vi "ASK.vi"() -> ()   [LabVIEW 2015]
panel:
  out "modulated":dbl[](graph)
  out "carrier":dbl[](graph)
  out "data":i16[](graph)
  in  "Carrier Frequency":dbl
  in  "Numeric":i32
  in  "Sampling Frequency":i32
  in  "data Frequency":dbl
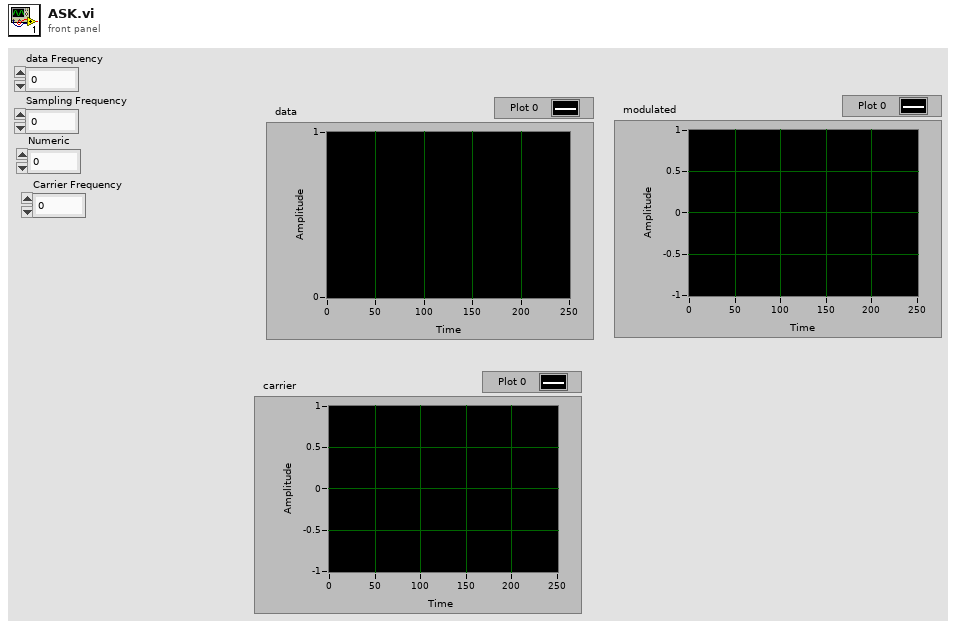
[diagram p1: front panel]
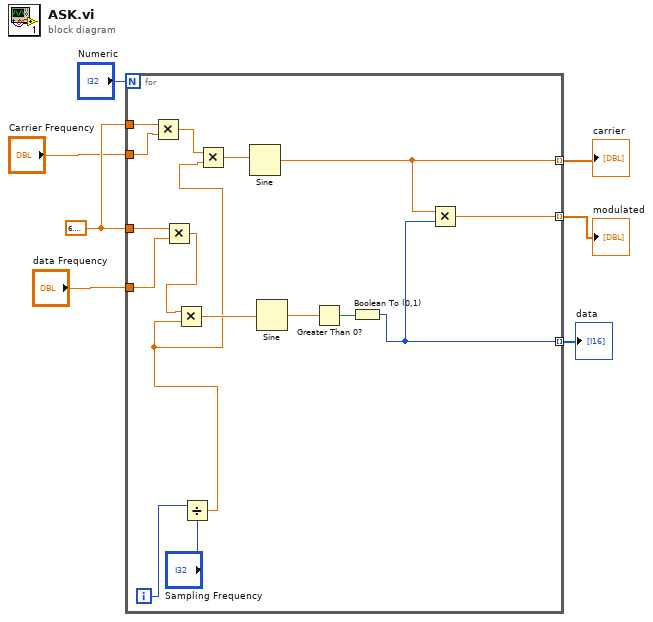
[diagram p0: block diagram]
diagram:
  w5 = 6.283185307179586
  n1 = for {
    N: "Numeric" -> [_]
    tunnel: w5 -> [w23]
    tunnel: "data Frequency" -> [w22]
    tunnel: w5 -> [w17]
    tunnel: "Carrier Frequency" -> [w16]
    tunnel: [w9] -> w3 mode=indexing
    tunnel: [w10] -> w2 mode=indexing
    tunnel: [w8] -> w1 mode=indexing
    i -> [w21]
    n2 = Multiply(x=w17, y=w16) -> (x*y=w15:dbl)
    n3 = Multiply(x=w23, y=w22) -> (x*y=w19:dbl)
    n4 = Divide(x=w21, y="Sampling Frequency") -> (x/y=w14:dbl)
    n5 = Multiply(x=w19, y=w14) -> (x*y=w18:dbl)
    n6 = Multiply(x=w15, y=w14) -> (x*y=w13:dbl)
    n7 = Sine(x=w13) -> (sin(x)=w10:dbl)
    n8 = Sine(x=w18) -> (sin(x)=w11:dbl)
    n9 = Greater Than 0?(x=w11) -> (x > 0?=w12:bool)
    n10 = Boolean To (0,1)(Boolean=w12) -> (0, 1=w9:i16)
    n11 = Multiply(x=w10, y=w9) -> (x*y=w8:dbl)
  }
  "data" <- w3
  "carrier" <- w2
  "modulated" <- w1
